vi "Define.vi"(11 "Definition":T1) -> (3 "Text out":refnum<class "Text.lvclass">)   [LabVIEW 2020, in "Conditum.lvlib" / "Columns.lvlib" / "Text.lvclass"]
uses:
  Text.lvclass
  Type/Type.lvclass
  LabVIEW Type.ctl
  Conditum.lvlib
  Type/Definition.ctl
  Definition.ctl
  Text Definition.ctl
  Attributes.ctl
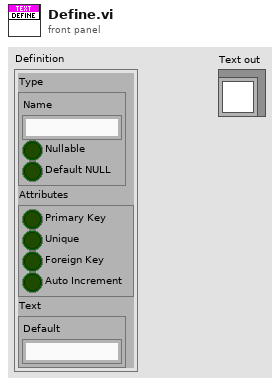
[diagram p1: front panel]
types:
  T1 = typedef "Conditum.lvlib/Columns.lvlib/Text.lvclass/Text Definition.ctl" = cluster{"Type":T2, "Attributes":T3, "Text":T4}
  T2 = typedef "Conditum.lvlib/Columns.lvlib/Type.lvclass/Definition.ctl" = cluster{"Name":string, "Nullable":bool, "Default NULL":bool}
  T3 = typedef "Conditum.lvlib/Attributes.ctl" = cluster{"Primary Key":bool, "Unique":bool, "Foreign Key":bool, "Auto Increment":bool}
  T4 = typedef "Conditum.lvlib/Columns.lvlib/Text.lvclass/Definition.ctl" = cluster{"Default":string}
  T5 = typedef "Conditum.lvlib/LabVIEW Type.ctl" = enum16{"None", "ID", "Boolean", "Integer", "Double", "Timestamp", "String", "Text", "Entity"}
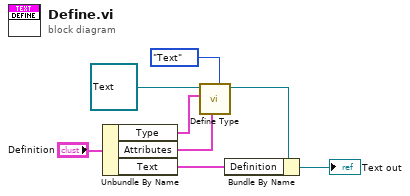
[diagram p0: block diagram]
diagram:
  n1 = Unbundle By Name("Definition") -> ("Type"=w6:T2, "Attributes"=w2:T3, "Text"=w5:T4)
  n2 = call "Define Type.vi"("Type"=LabVIEW_Type."Text", "Attributes"=w2, "Definition"=w6, "Type in"=refnum<class "Text.lvclass"> refnum ("Text out")) -> ("Type out"=w4:refnum<class "Text.lvclass">)  [unwired: 7 in]
  n3 = Bundle By Name(cluster=w4, "Definition"=w5) -> (→"Text out":refnum<class "Text.lvclass">)
